vi "Analysis.Result Summaries, Generate Pareto comparing Locations_V2.vi"(11 "ResultSum":T1[](array[typedef])) -> (0 "Fault% Per Station":cluster{i32[], dbl[]}[](array[cluster]), 1 "Station Names":string[](array[string]), 2 "FaultCodes":string[](array[string]), 3 "Location Yield Comparison Table_%":string[][](table), 5 "Location Yield Comparison Table_Cnts":string[][](table))   [LabVIEW 2024]
uses:
  Analysis.Station Fail Paredo Gen Input_V2.ctl
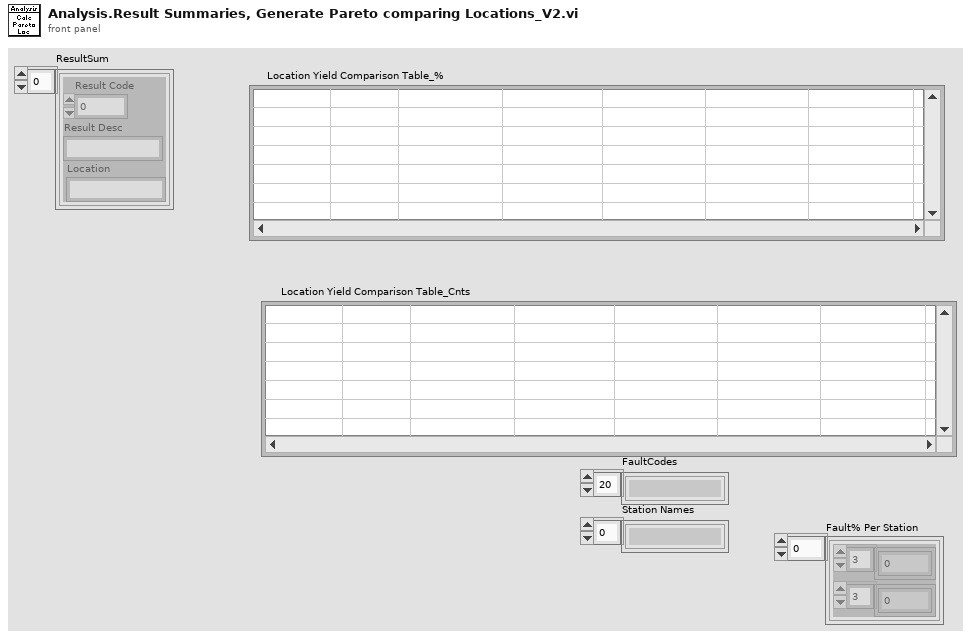
[diagram p1: front panel]
types:
  T1 = typedef "Analysis.Station Fail Paredo Gen Input_V2.ctl" = cluster{"Result Code":i32, "Result Desc":string, "Location":string}
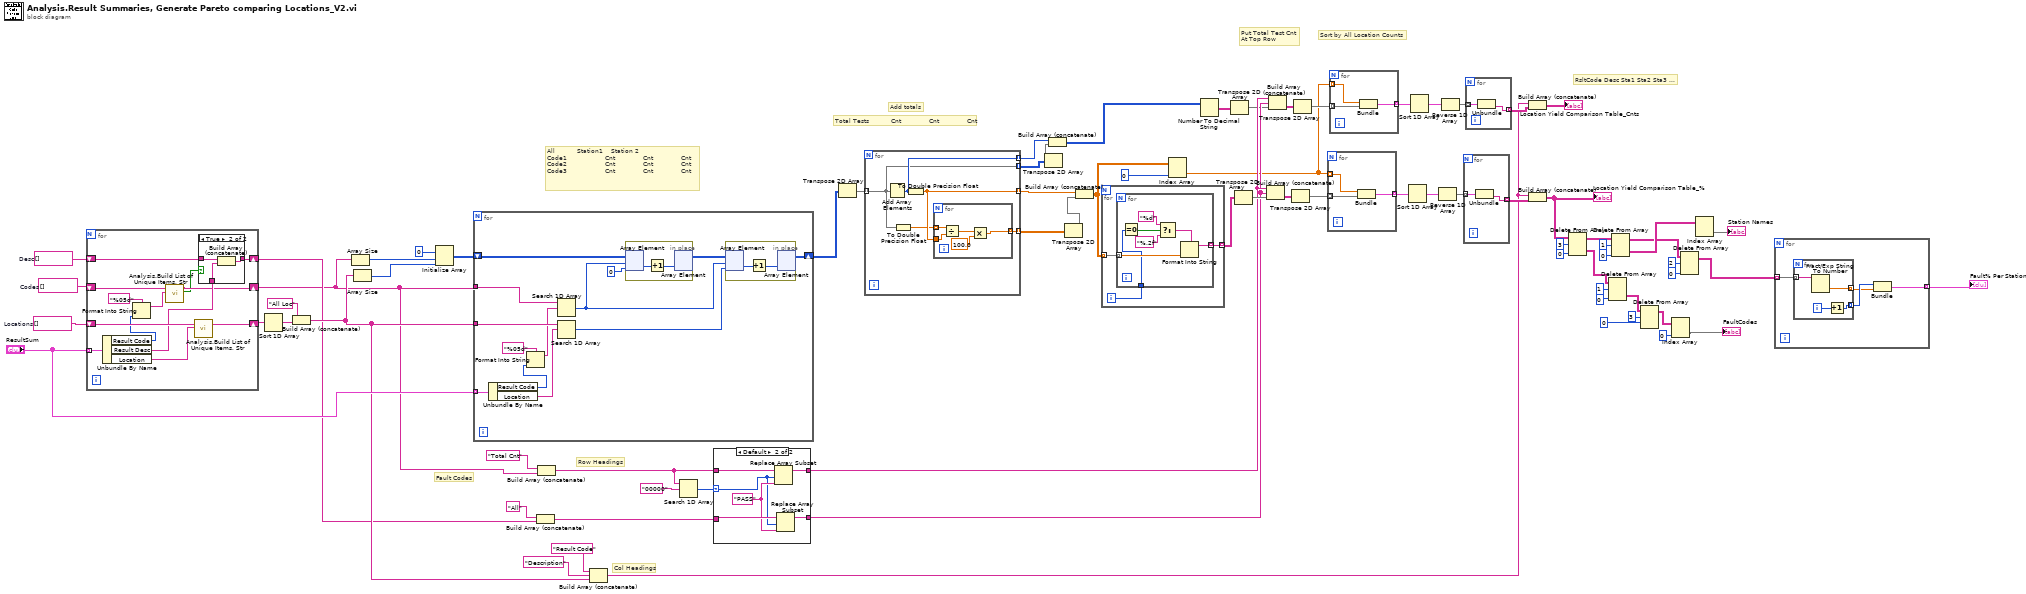
[diagram p0: block diagram]
diagram:
  w26 = string[] []  # Desc
  w75 = string[] []  # Codes
  w76 = string[] []  # Locations
  # "RsltCode Desc Sta1 Sta2 Sta3 ..."
  # "Fault Codes"
  # "Put Total Test Cnt\nAt Top Row"
  # "Sort by All Location Counts"
  # "Col Headings"
  # "Row Headings"
  # "Add totals"
  # "Total Tests           Cnt              Cnt              Cnt"
  # "All           Station1    Station 2   \nCode1                   Cnt              Cnt              Cnt\nCode2                   Cnt              Cnt              Cnt\nCode3                   Cnt              Cnt              Cnt"
  n1 = for {
    shift-right: [w88] -> w58
    shift-left: w76 -> [w89]
    shift-right: [w81] -> w19
    shift-left: w75 -> [w82]
    tunnel: "ResultSum" -> [w87] mode=indexing
    shift-right: [w83] -> w22
    shift-left: w26 -> [w84]
    n2 = Unbundle By Name(w87) -> ("Result Code"=w77:i32, "Result Desc"=w85:string, "Location"=w86:string)
    n3 = Format Into String(format string="%05d", w77) -> (resulting string=w78:string)  [unwired: 2 in, 1 out]
    n4 = call "Analysis.Build List of Unique Items, Str.vi"("Item In"=w78, "List In"=w82) -> ("Added"=w80:bool, "List Out"=w81:string[])  [unwired: 7 in, 1 out]
    n5 = call "Analysis.Build List of Unique Items, Str.vi"("Item In"=w86, "List In"=w89) -> ("List Out"=w88:string[])  [unwired: 7 in, 2 out]
    n6 = case shown="True" w80 {
      tunnel: w85 -> [_ w91]
      tunnel: w84 -> [w90 w93]
      tunnel: [w90 w92] -> w83
      frame False {
      }
      frame True {
        n7 = Build Array (concatenate)(w93, w91) -> (w92:string[])
      }
    }
  }
  n8 = Sort 1D Array(array=w58) -> (sorted array=w57:string[])
  n9 = Build Array (concatenate)("All Loc" ("String"), w57) -> (w55:string[])
  n10 = Array Size(array=w19) -> (size(s)=w71:i32)
  n11 = Array Size(array=w55) -> (size(s)=w70:i32)
  n12 = Initialize Array(0, w71, w70) -> (w73:i32[][])
  n13 = for {
    shift-right: [w100] -> w68
    shift-left: w73 -> [w102]
    tunnel: "ResultSum" -> [w106] mode=indexing
    tunnel: w19 -> [w105]
    tunnel: w55 -> [w104]
    n14 = Unbundle By Name(w106) -> ("Result Code"=w95:i32, "Location"=w103:string)
    n15 = Format Into String(format string="%05d", w95) -> (resulting string=w94:string)  [unwired: 2 in, 1 out]
    n16 = Search 1D Array(1D array=w105, element=w94) -> (index of element=w99:i32)  [unwired: 1 in]
    n17 = Search 1D Array(1D array=w104, element=w103) -> (index of element=w97:i32)  [unwired: 1 in]
    n18 = in-place {
      n19 = in-place-array #1(w102, w99, 0) -> (w110:i32)
      n20 = Increment(x=w110) -> (x+1=w109:i32)
      n21 = in-place-array #1(w109) -> (w101:i32[][])  [unwired: 2 out]
    }
    n22 = in-place {
      n23 = in-place-array #2(w101, w99, w97) -> (w108:i32)
      n24 = Increment(x=w108) -> (x+1=w107:i32)
      n25 = in-place-array #2(w107) -> (w100:i32[][])  [unwired: 2 out]
    }
  }
  n26 = Build Array (concatenate)("All", w22) -> (w21:string[])
  n27 = Build Array (concatenate)("Total Cnt", w19) -> (w53:string[])
  n28 = Build Array (concatenate)("Result Code", "Description", w55) -> (w5:string[])
  n29 = Search 1D Array(1D array=w53, element="00000") -> (index of element=w52:i32)  [unwired: 1 in]
  n30 = case shown="Default" w52 {
    selector: w52 -> [_ w114]
    tunnel: w53 -> [w112 w118]
    tunnel: [w112 w117] -> w9
    tunnel: w21 -> [w111 w116]
    tunnel: [w111 w113] -> w8
    frame -1 {
    }
    frame Default {
      w115 = "PASS" ("new element/subarray")
      n31 = Replace Array Subset(array=w118, new element=w115, index=w114) -> (w117:string[])
      n32 = Replace Array Subset(array=w116, new element=w115, index=w114) -> (w113:string[])
    }
  }
  n33 = Transpose 2D Array(2D array=w68) -> (transposed array=w69:i32[][])
  n34 = for {
    tunnel: w69 -> [w119] mode=indexing
    tunnel: [w122] -> w18 mode=indexing
    tunnel: [w123] -> w51 mode=indexing
    tunnel: [w120] -> w15 mode=indexing
    tunnel: [w119] -> w16 mode=indexing
    n35 = Add Array Elements(numeric array=w119) -> (sum=w120:i32)
    n36 = To Double Precision Float(number=w119) -> (double precision float=w121:dbl[])
    n37 = To Double Precision Float(number=w120) -> (double precision float=w122:dbl)
    n38 = for {
      tunnel: w121 -> [w128] mode=indexing
      tunnel: w122 -> [w127]
      tunnel: [w124] -> w123 mode=indexing
      n39 = Divide(x=w128, y=w127) -> (x/y=w126:dbl)
      n40 = Multiply(x=w126, y=100.0) -> (x*y=w124:dbl)
    }
  }
  n41 = Transpose 2D Array(2D array=w16) -> (transposed array=w17:i32[][])
  n42 = Build Array (concatenate)(w15, w17) -> (w2:i32[][])
  n43 = Transpose 2D Array(2D array=w51) -> (transposed array=w50:dbl[][])
  n44 = Build Array (concatenate)(w18, w50) -> (w49:dbl[][])
  n45 = for {
    tunnel: w49 -> [w131] mode=indexing
    tunnel: [w130] -> w48 mode=indexing
    i -> [w129]
    n46 = for {
      tunnel: w131 -> [w138] mode=indexing
      tunnel: [w137] -> w130 mode=indexing
      tunnel: w129 -> [w132]
      n47 = Equal To 0?(x=w132) -> (x = 0?=w133:bool)
      n48 = Select(t="%d" ("format string"), s=w133, f="%.2f" ("format string")) -> (s? t:f=w136:string)
      n49 = Format Into String(format string=w136, w138) -> (resulting string=w137:string)  [unwired: 2 in, 1 out]
    }
  }
  n50 = Index Array(array=w49, index (col)=0 ("disabled index (col)")) -> (element=w7:dbl[])  [unwired: 1 in]
  n51 = Number To Decimal String(number=w2) -> (decimal integer string=w1:string[][])  [unwired: 1 in]
  n52 = Transpose 2D Array(2D array=w1) -> (transposed array=w3:string[][])
  n53 = Transpose 2D Array(2D array=w48) -> (transposed array=w66:string[][])
  n54 = Build Array (concatenate)(w9, w8, w66) -> (w65:string[][])
  n55 = Build Array (concatenate)(w9, w8, w3) -> (w10:string[][])
  n56 = Transpose 2D Array(2D array=w65) -> (transposed array=w64:string[][])
  n57 = Transpose 2D Array(2D array=w10) -> (transposed array=w11:string[][])
  n58 = for {
    tunnel: w64 -> [w141] mode=indexing
    tunnel: w7 -> [w140] mode=indexing
    tunnel: [w139] -> w63 mode=indexing
    n59 = Bundle(w140, w141) -> (w139:cluster{dbl, string[]})  [unwired: 1 in]
  }
  n60 = for {
    tunnel: w11 -> [w144] mode=indexing
    tunnel: w7 -> [w143] mode=indexing
    tunnel: [w142] -> w12 mode=indexing
    n61 = Bundle(w143, w144) -> (w142:cluster{dbl, string[]})  [unwired: 1 in]
  }
  n62 = Sort 1D Array(array=w63) -> (sorted array=w62:cluster{dbl, string[]}[])
  n63 = Sort 1D Array(array=w12) -> (sorted array=w13:cluster{dbl, string[]}[])
  n64 = Reverse 1D Array(array=w62) -> (reversed array=w61:cluster{dbl, string[]}[])
  n65 = Reverse 1D Array(array=w13) -> (reversed array=w14:cluster{dbl, string[]}[])
  n66 = for {
    tunnel: w61 -> [w146] mode=indexing
    tunnel: [w145] -> w60 mode=indexing
    n67 = Unbundle(w146) -> (w145:string[])  [unwired: 1 out]
  }
  n68 = for {
    tunnel: w14 -> [w148] mode=indexing
    tunnel: [w147] -> w6 mode=indexing
    n69 = Unbundle(w148) -> (w147:string[])  [unwired: 1 out]
  }
  n70 = Build Array (concatenate)(w5, w6) -> (→"Location Yield Comparison Table_Cnts":string[][])
  n71 = Build Array (concatenate)(w5, w60) -> (w20:string[][])
  "Location Yield Comparison Table_%" <- w20
  n72 = Delete From Array(array=w20, length=3, index (col)=0 ("disabled index (col)")) -> (deleted portion=w39:string[][], array with subset deleted=w45:string[][])  [unwired: 1 in]
  n73 = Delete From Array(array=w39, length=1, index (col)=0 ("index (row)")) -> (deleted portion=w37:string[][])  [unwired: 1 in, 1 out]
  n74 = Delete From Array(array=w45, length=1, index (row)=0) -> (deleted portion=w42:string[][], array with subset deleted=w31:string[][])  [unwired: 1 in]
  n75 = Delete From Array(array=w37, length=3, index (row)=0) -> (array with subset deleted=w30:string[][])  [unwired: 1 in, 1 out]
  n76 = Index Array(array=w30, index (col)=0 ("disabled index (col)")) -> (element=→"FaultCodes":string[])  [unwired: 1 in]
  n77 = Delete From Array(array=w31, length=2, index (row)=0) -> (array with subset deleted=w28:string[][])  [unwired: 1 in, 1 out]
  n78 = Index Array(array=w42) -> (element=→"Station Names":string[])  [unwired: 2 in]
  n79 = for {
    tunnel: w28 -> [w150] mode=indexing
    tunnel: [w149] -> w27 mode=indexing
    n80 = for {
      tunnel: w150 -> [w156] mode=indexing
      tunnel: [w155] -> w151 mode=indexing
      tunnel: [w153] -> w152 mode=indexing
      i -> [w154]
      n81 = Fract/Exp String To Number(string=w156) -> (number=w155:dbl)  [unwired: 3 in, 1 out]
      n82 = Increment(x=w154) -> (x+1=w153:i32)
    }
    n83 = Bundle(w152, w151) -> (w149:cluster{i32[], dbl[]})  [unwired: 1 in]
  }
  "Fault% Per Station" <- w27
